vi "Close.vi"(8 "error in (no error)":errorcluster, 11 "reference in":refnum<class "Medulla_ATE.lvclass">) -> (0 "error out":errorcluster, 3 "reference in":refnum<class "Medulla_ATE.lvclass">)   [LabVIEW 2022 SP3, in "Medulla_ATE.lvlib" / "Medulla_ATE.lvclass"]
uses:
  Medulla_ATE.lvclass
  Components/ViPER.lvlibp/ViPER.lvclass
  C:/Projects/Medulla/ViPER/Examples/Flux_Capacitor_Tester/Components/ViPER.lvlibp/ViPER.lvclass
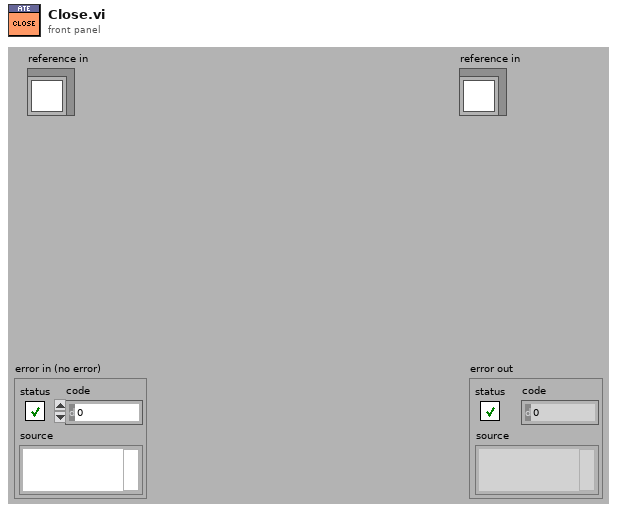
[diagram p1: front panel]
types:
  T1 = typedef "Medulla_ATE.lvlib/Medulla_ATE.lvclass/ObjectAttributes.ctl" = cluster{"Config":T2, "DUT_Handler":refnum<class "DUT_Handler_Base.lvclass">, "MES":refnum<class "MES_Base.lvclass">, "TestView":refnum<class "TestView_Base.lvclass">, "TestClass":refnum<class "Test_Base.lvclass">}
  T2 = typedef "Medulla_ATE.lvlib/Medulla_ATE.lvclass/Config.ctl" = cluster{"ForceStart":bool, "ForceAbort":bool}
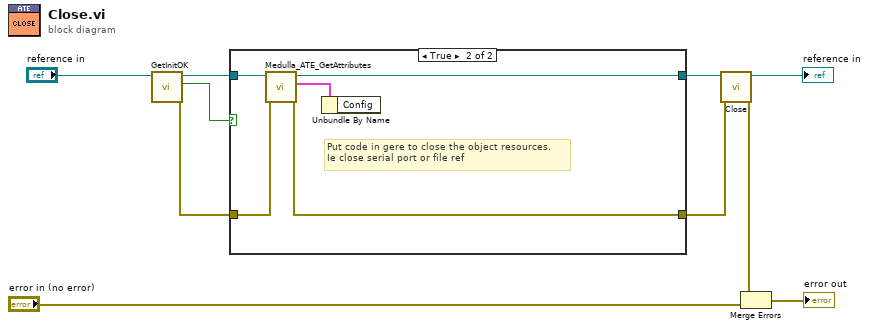
[diagram p0: block diagram]
diagram:
  n1 = call "GetInitOK.vi"("reference in"="reference in") -> ("error out"=w4:errorcluster, "init_ok"=w5:bool, "reference out"=w6:refnum<class "Medulla_ATE.lvclass">)  [unwired: 8 in]
  n2 = case shown="True" w5 {
    tunnel: w4 -> [w12 w16]
    tunnel: [w12 w15] -> w7
    tunnel: w6 -> [w11 w17]
    tunnel: [w11 w13] -> w8
    frame False {
    }
    frame True {
      # "Put code in gere to close the object resources.\nIe close serial port or file ref"
      n3 = call "Medulla_ATE_GetAttributes.vi"("error in (no error)"=w16, "reference in"=w17) -> ("error out"=w15:errorcluster, "Data"=w14:T1, "reference out"=w13:refnum<class "Medulla_ATE.lvclass">)  [unwired: 6 in, 1 out]
      n4 = Unbundle By Name(w14) -> ()  [unwired: 1 out]
    }
  }
  n5 = call-parent "Close.vi"("error in (no error)"=w7, "reference in"=w8) -> ("error out"=w3:errorcluster, "reference out"=→"reference in":refnum<class "Medulla_ATE.lvclass">)  [unwired: 8 in]
  n6 = Merge Errors(w3, "error in (no error)") -> (→"error out":errorcluster)
